vi "deltaPS.vi"(11 "VISA resource name":refnum<visa-resource-name>) -> ()   [LabVIEW 2019]
uses:
  DELTA ELEKTRONIKA SM Series/DELTA ELEKTRONIKA.lvlib
panel:
  in  "Stop Main":bool
  out "Actual Voltage Level (V)":dbl format="%.2f"
  out "Actual Current Limit (A)":dbl format="%.2f"
  out "Voltage Limit":bool
  out "Current Limit":bool
  in  "Voltage Level (0.0 V)":dbl format="%.2f"
  in  "Current Limit (0A)":dbl format="%.2f"
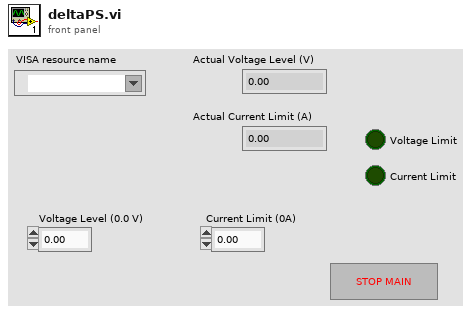
[diagram p1: front panel]
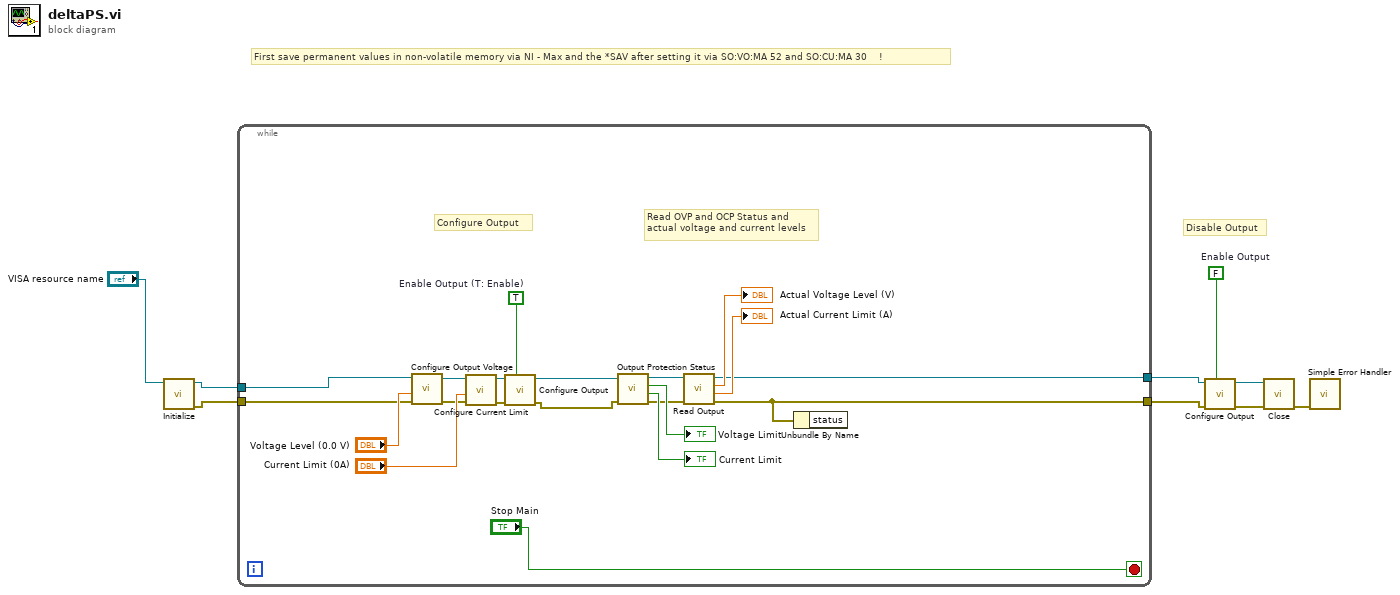
[diagram p0: block diagram]
diagram:
  w3 = FALSE  # Enable Output
  # "Disable Output"
  # "First save permanent values in non-volatile memory via NI - Max and the *SAV after setting it via SO:VO:MA 52 and SO:CU:MA 30    !"
  n1 = call "Initialize.vi"("VISA resource name"="VISA resource name") -> ("error out"=w8:errorcluster, "VISA resource name out"=w7:refnum<visa-resource-name>)  [unwired: 9 in]
  n2 = while {
    tunnel: w8 -> [w22]
    tunnel: w7 -> [w21]
    tunnel: [w11] -> w2
    tunnel: [w10] -> w1
    stop <- "Stop Main" stop-if-true
    w26 = TRUE  # Enable Output (T: Enable)
    # "Read OVP and OCP Status and\nactual voltage and current levels"
    # "Configure Output"
    n3 = call "Configure Output Voltage.vi"("error in (no error)"=w22, "Set Voltage(0.0 V)"="Voltage Level (0.0 V)", "VISA resource name"=w21) -> ("error out"=w25:errorcluster, "VISA resource name out"=w24:refnum<visa-resource-name>)  [unwired: 7 in]
    n4 = call "Configure Current Limit.vi"("error in (no error)"=w25, "Current Limit (0.0 A)"="Current Limit (0A)", "VISA resource name"=w24) -> ("error out"=w28:errorcluster, "VISA resource name out"=w29:refnum<visa-resource-name>)  [unwired: 7 in]
    n5 = call "Configure Output.vi"("Enable Output (T: Enable)"=w26, "error in (no error)"=w28, "VISA resource name"=w29) -> ("error out"=w13:errorcluster, "VISA resource name out"=w12:refnum<visa-resource-name>)  [unwired: 7 in]
    n6 = call "Output Protection Status.vi"("error in (no error)"=w13, "VISA resource name"=w12) -> ("error out"=w15:errorcluster, "OCP Tripped?"=→"Current Limit":bool, "OVP Tripped?"=→"Voltage Limit":bool, "VISA resource name out"=w14:refnum<visa-resource-name>)  [unwired: 6 in]
    n7 = call "Read Output.vi"("error in (no error)"=w15, "VISA resource name"=w14) -> ("error out"=w10:errorcluster, "Actual Current Level (A)"=→"Actual Current Limit (A)":dbl, "Actual Voltage Level (V)"=→"Actual Voltage Level (V)":dbl, "VISA resource name out"=w11:refnum<visa-resource-name>)  [unwired: 6 in]
    n8 = Unbundle By Name(w10) -> ()  [unwired: 1 out]
  }
  n9 = call "Configure Output.vi"("Enable Output (T: Enable)"=w3, "error in (no error)"=w1, "VISA resource name"=w2) -> ("error out"=w5:errorcluster, "VISA resource name out"=w4:refnum<visa-resource-name>)  [unwired: 7 in]
  n10 = call "Close.vi"("error in (no error)"=w5, "VISA resource name"=w4) -> ("error out"=w6:errorcluster)  [unwired: 9 in]
  n11 = call <vilib>:"Simple Error Handler.vi"("error in (no error)"=w6) -> ()  [unwired: 4 in, 5 out]
